vi "U3 Pin Configuration Example.vi"() -> (0 "error out":errorcluster)   [LabVIEW 2021]
panel:
  in  "Set Defaults":bool
  in  "EIO Analog Enable":bool[](array[boolean])=[FALSE, FALSE, FALSE, FALSE, FALSE, FALSE, FALSE, FALSE]
  in  "FIO Analog Enable":bool[](array[boolean])=[FALSE, FALSE, FALSE, FALSE, FALSE, FALSE, FALSE, FALSE]
  in  "Timer/Counter Pin Offset":u8
  in  "Enable Counter1":bool
  in  "Enable Counter0":bool
  in  "Enable DAC1":bool
  in  "Number of Timers Enabled":u8
  in  "FirstFound":bool=TRUE
  in  "Address":string="1"
  out "Error Message":string
  # "Reads 1 input or writes 1 output.  Use \"U3 Pin Configuration Example.vi\" to set pins to digital\nor analog."
  # "This causes the current pin configuration\nto become the new power-up default.\nThis is done by writing the values\nto flash, and flash memory has a limited\nlifetime (~20k writes), so we have hidden\nthe continuous run button in the LabVIEW\ntoolbar for this VI."
  # "0"
  # "1"
  # "2"
  # "3"
  # "4"
  # "5"
  # "6"
  # "7"
  # "8"
  # "9"
  # "10"
  # "11"
  # "12"
  # "13"
  # "14"
  # "15"
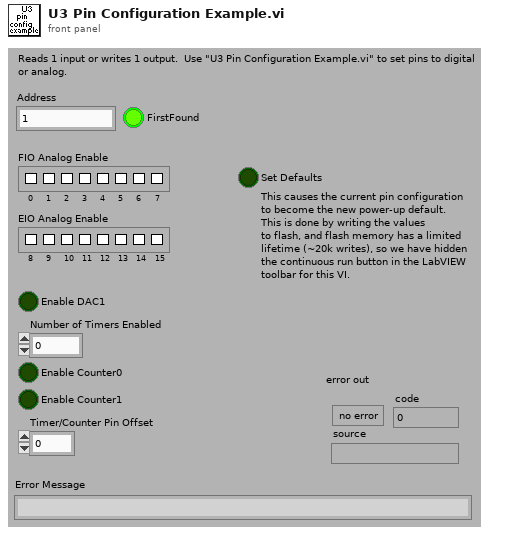
[diagram p1: front panel]
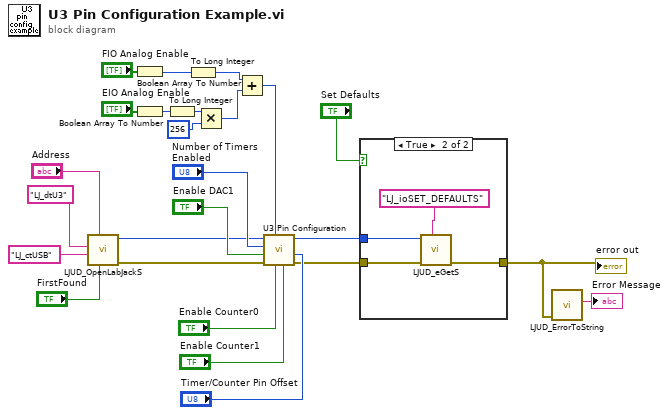
[diagram p0: block diagram]
diagram:
  n1 = call "LJUD_OpenLabJackS.vi"("FirstFound"="FirstFound", "Address"="Address", "ConnectionType"="LJ_ctUSB", "DeviceType"="LJ_dtU3") -> ("error out"=w14:errorcluster, "Handle"=w15:i32)  [unwired: 5 in, 1 out]
  n2 = Boolean Array To Number(Boolean array="FIO Analog Enable") -> (number=w3:u32)
  n3 = Boolean Array To Number(Boolean array="EIO Analog Enable") -> (number=w2:u32)
  n4 = To Long Integer(number=w2) -> (32bit integer=w5:i32)
  n5 = To Long Integer(number=w3) -> (32bit integer=w6:i32)
  n6 = Multiply(x=w5, y=256) -> (x*y=w4:i32)
  n7 = Add(x=w6, y=w4) -> (x+y=w1:i32)
  n8 = call "U3 Pin Configuration.vi"("Timer/Counter Pin Offset"="Timer/Counter Pin Offset", "Enable Counter1"="Enable Counter1", "Enable Counter0"="Enable Counter0", "FIO/EIO Analog Enable"=w1, "error in"=w14, "Enable DAC1"="Enable DAC1", "Number of Timers Enabled"="Number of Timers Enabled", "Handle In"=w15) -> ("error out"=w11:errorcluster, "Handle Out"=w10:i32)  [unwired: 2 in]
  n9 = case shown="True" "Set Defaults" {
    tunnel: w11 -> [w26 w30]
    tunnel: w10 -> [_ w29]
    tunnel: [w26 w27] -> w9
    frame False {
    }
    frame True {
      n10 = call "LJUD_eGetS.vi"("IOType"="LJ_ioSET_DEFAULTS", "error in"=w30, "Handle In"=w29) -> ("error out"=w27:errorcluster)  [unwired: 6 in, 2 out]
    }
  }
  "error out" <- w9
  n11 = call "LJUD_ErrorToString.vi"("error in"=w9) -> ("String"=→"Error Message":string)  [unwired: 10 in]
